vi "ITC IL test.vi"() -> ()   [LabVIEW 2013, in "Mercury iXX.lvlib"]
uses:
  <instrlib>/Mercury iXX/Mercury iXX.lvlib
  <instrlib>/Mercury iXX/Public/Controls/Comms Transport Layer.ctl
  <instrlib>/Mercury iXX/Public/Controls/Serial Settings.ctl
  <instrlib>/Mercury iXX/Public/Controls/ISOBus Address.ctl
panel:
  out "Ch Info":T1(array[cluster])
  out "error out":errorcluster
  out "Device Details":T2
  in  "Interval between messages (ms)":i16=10
  in  "stop":bool
  in  "Connection Details":T6={"VISA resource name"="", "Comms Layer"=enum."Ethernet TCP/IP", "IP Address"="", "Serial Configuration"={"Baud Rate"=115200, "Parity"=0, "Data Bits"=8, "Stop Bits"=10, "Flow Control"=0}, "ISOBUS address"=-1} {"Serial Configuration"."Flow Control" items=["None", "XON/XOFF", "RTS/CTS", "XON/XOFF & RTS/CTS", "DTR/DSR", "XON/XOFF & DTR/DSR"]; "Serial Configuration"."Stop Bits" items=["1.0"=10, "2.0"=20]; "Serial Configuration"."Data Bits" items=["7"=7, "8"=8]; "Serial Configuration"."Parity" items=["None", "Odd", "Even"]; "Serial Configuration"."Baud Rate" items=["300"=300, "600"=600, "1200"=1200, "2400"=2400, "4800"=4800, "9600"=9600, "14400"=14400, "19200"=19200, "38400"=38400, "57600"=57600, "115200"=115200]}
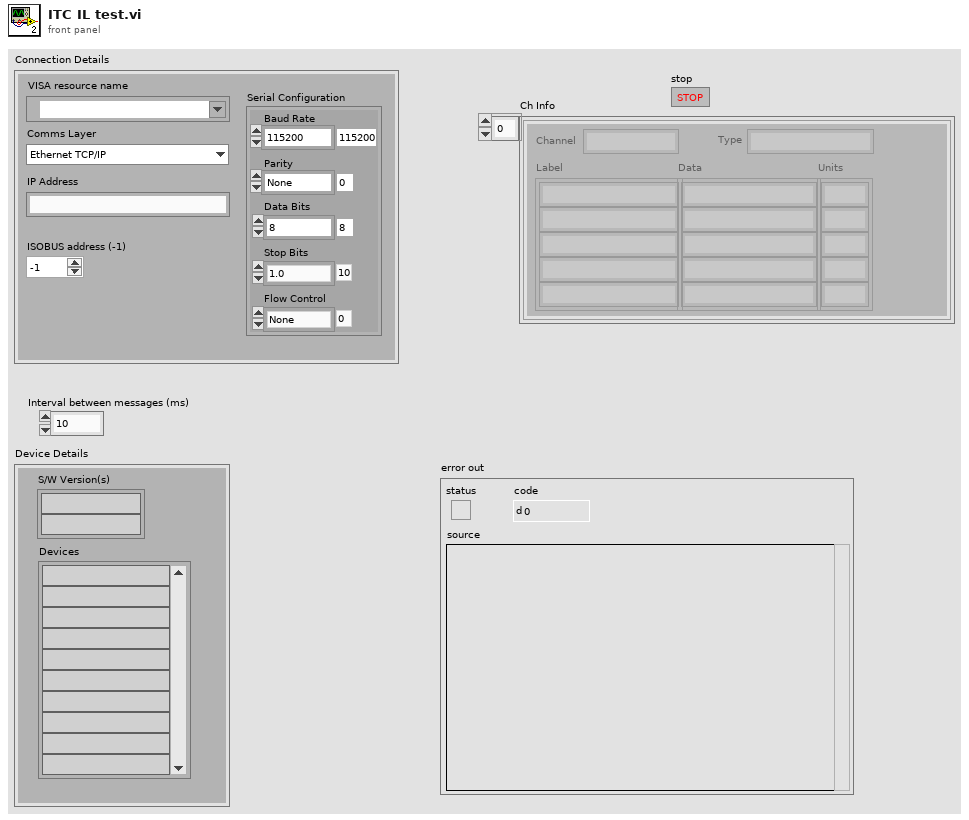
[diagram p1: front panel]
types:
  T1 = cluster{"Data":string[], "Label":string[], "Units":string[], "Channel":string, "Type":string}[]
  T2 = cluster{"Devices":string[], "S/W Version(s)":string[]}
  T3 = typedef "Mercury iXX.lvlib/Comms Transport Layer.ctl" = enum16{"Ethernet TCP/IP", "USB", "ISOBus - RS-232", "GPIB"}
  T4 = typedef "Mercury iXX.lvlib/Serial Settings.ctl" = cluster{"Baud Rate":u32, "Parity":u16, "Data Bits":u16, "Stop Bits":u16, "Flow Control":u16}
  T5 = typedef "Mercury iXX.lvlib/ISOBus Address.ctl" = i32
  T6 = cluster{"VISA resource name":refnum<visa-resource-name>, "Comms Layer":T3, "IP Address":string, "Serial Configuration":T4, "ISOBUS address":T5}
  T7 = typedef "Mercury iXX.lvlib/Mercury Reference.ctl" = cluster{"Comms":refnum<visa-resource-name>, "Device ID":string[], "Comms Layer":T3, "Command":string, "Query reference":T8}
  T8 = typedef "Mercury iXX.lvlib/Query Dynamic Reference.ctl" = refnum<vi>
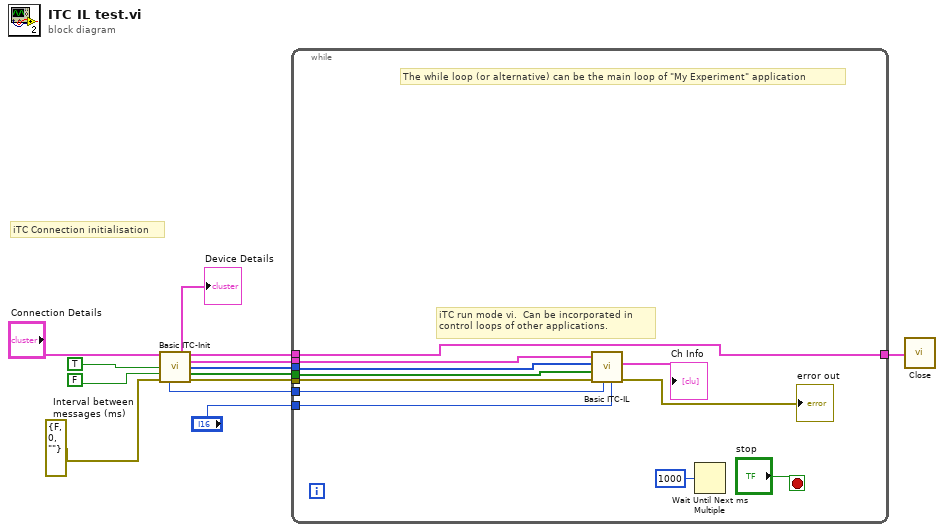
[diagram p0: block diagram]
diagram:
  # "iTC Connection initialisation"
  n1 = call <instrlib>:"Basic ITC-Init.vi"("Connection Details"="Connection Details", "ID Query (True)"=TRUE, "Clear Previous Connections (False)"=FALSE, "error in (no error)"=errorcluster {"status"=FALSE, "code"=0, "source"=""}) -> ("Device Details"=→"Device Details":T2, "Merc Ref Out"=w12:T7, "Device_ref_Array"=w11:T7[], "Ch_type_index"=w10:i32[], "Device_Present?"=w7:bool[], "ISOBUS address"=w8:T5, "error out"=w9:errorcluster)  [unwired: 5 in]
  n2 = while {
    tunnel: "Interval between messages (ms)" -> [w21]
    tunnel: w12 -> [w22]
    tunnel: w11 -> [w16]
    tunnel: w10 -> [w17]
    tunnel: w9 -> [w20]
    tunnel: w8 -> [w19]
    tunnel: w7 -> [w18]
    tunnel: [w22] -> w6
    stop <- "stop" stop-if-true
    # "iTC run mode vi.  Can be incorporated in\ncontrol loops of other applications."
    # "The while loop (or alternative) can be the main loop of \"My Experiment\" application"
    n3 = call <instrlib>:"Basic ITC-IL.vi"("Interval between messages (ms)"=w21, "ISOBUS address"=w19, "error in (no error)"=w20, "Device_Present?"=w18, "Ch_type_index"=w17, "Merc_ref_Array"=w16) -> ("error out"=→"error out":errorcluster, "Ch Info"=→"Ch Info":T1)  [unwired: 2 in]
    n4 = Wait Until Next ms Multiple(millisecond multiple=u32 1000) -> ()  [unwired: 1 out]
  }
  n5 = call <instrlib>:"Close.vi"("Mercury Reference"=w6) -> ()  [unwired: 10 in, 1 out]
